vi "Untitled 1.vi"() -> ()   [LabVIEW 2018]
panel:
  out "Boolean 4":bool
  out "Boolean 3":bool
  in  "Boolean 2":bool
  in  "Boolean":bool
  out "Numeric 4":dbl
  in  "Numeric 3":dbl
  in  "Numeric 2":dbl
  in  "Numeric":dbl
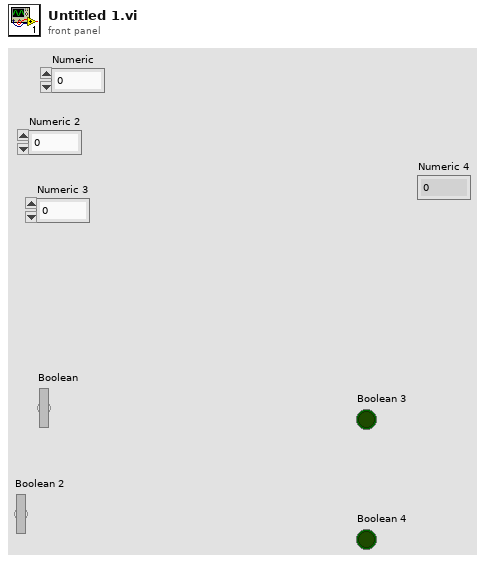
[diagram p1: front panel]
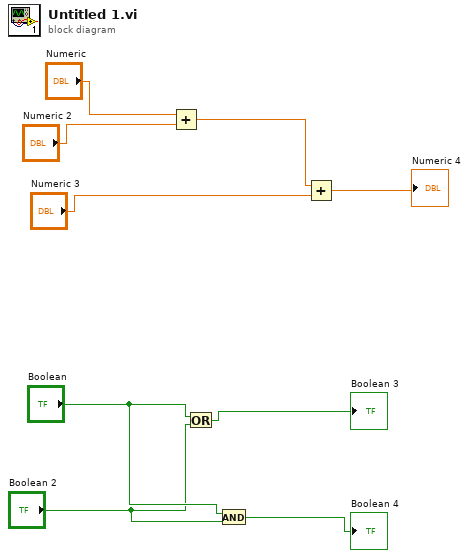
[diagram p0: block diagram]
diagram:
  n1 = Add(x="Numeric", y="Numeric 2") -> (x+y=w6:dbl)
  n2 = Or(x="Boolean", y="Boolean 2") -> (x .or. y?=→"Boolean 3":bool)
  n3 = And(x="Boolean", y="Boolean 2") -> (x .and. y?=→"Boolean 4":bool)
  n4 = Add(x=w6, y="Numeric 3") -> (x+y=→"Numeric 4":dbl)
